vi "Init.vi"(8 "error in (no error)":errorcluster, 11 "Data in":refnum<class "OnChangeNotifier_I32.lvclass">) -> (0 "error out":errorcluster, 3 "Data out":refnum<class "OnChangeNotifier_I32.lvclass">)   [LabVIEW 2021, in "OnChangeNotifier_I32.lvclass"]
doc: "Abstract Data Classes 2.1.1.13\nTim Streeter - TSA\nCopyright (c) 2025, TSA"
uses:
  OnChangeNotifier_I32.lvclass
  C:/Program Files (x86)/National Instruments/LabVIEW 2021/vi.lib/TSA/Abstract Data Classes/Abs_Types/Value/Abs_Value.lvclass
  OnChangeNotifier_I32.lvclass/OnChangeNotifier_I32.ctl
  Properties/Read Data Type.vi
  Properties/Write Data Type.vi
  <vilib>/TSA/Abstract Data Classes/Abs_Types/I16 Integer/Abs_I16 Integer.lvclass
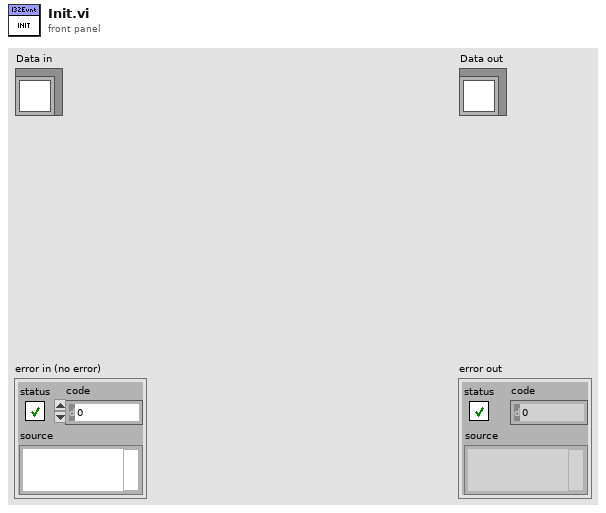
[diagram p1: front panel]
types:
  T1 = typedef "OnChangeNotifier_I32.lvclass/Class Type.ctl" = refnum<class "Abs_I16 Integer.lvclass">
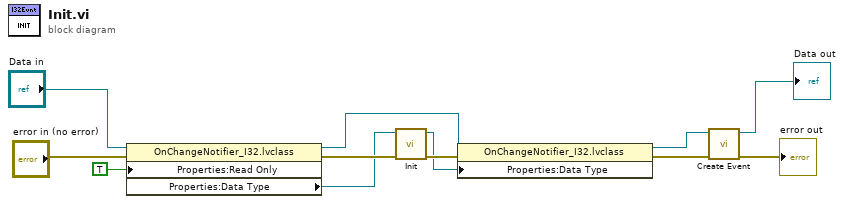
[diagram p0: block diagram]
diagram:
  n1 = property class="OnChangeNotifier_I32.lvclass"(reference="Data in", error in="error in (no error)", "Properties:Read Only"=TRUE ("Read Only")) -> (reference out=w7:refnum<class "OnChangeNotifier_I32.lvclass">, error out=w9:errorcluster, "Properties:Data Type"=w6:T1)
  n2 = call-dynamic "Init.vi"("error in (no error)"=w9, "Data in"=w6) -> ("error out"=w8:errorcluster, "Data out"=w5:T1)  [unwired: 8 in]
  n3 = property class="OnChangeNotifier_I32.lvclass"(reference=w7, error in=w8, "Properties:Data Type"=w5) -> (reference out=w2:refnum<class "OnChangeNotifier_I32.lvclass">, error out=w4:errorcluster)
  n4 = call-dynamic "Create Event.vi"("error in (no error)"=w4, "OnChange_Boolean in"=w2) -> ("error out"=→"error out":errorcluster, "OnChange_Boolean out"=→"Data out":refnum<class "OnChangeNotifier_I32.lvclass">)  [unwired: 8 in]
